vi "FinalizeScanSignals.vi"(8 "error in (no error)":errorcluster, 9 "Parameters":T1={"number of planes"=4, "z step"=1.9999999999999998e-05, "pixel dwell time"=1.0000000000000001e-11, "z frequency"=10.0, "number of pixels"=100, "smooth points"=10, "smooth line"=10, "Sine\nSawtooth"=FALSE, "PointSorting"=0, "Sort Points"=FALSE, "X-pixels"=256.0, "Y-lines"=256.0, "pixelstoµm"=256.0, "zoom"=1.0, "Time offset"=1.0000000000000001e-11} {"zoom" min=0.5 step=0.1; "Y-lines" min=1 step=1; "X-pixels" min=1 step=1; "PointSorting" items=["No Difference", "Every Second Point", "Down / Up"]; "smooth line" min=1; "smooth points" min=1; "number of pixels" min=1; "z frequency" format="%_4g"; "number of planes" min=1}, 10 "DutyCluster":T2 {"Iteration" items=["first iteration", "second iteration"]}, 11 "x pixels, y pixels, z, time":dbl[][](array[numeric])) -> (0 "error out":errorcluster, 3 "x (pixels), y (pixels), z (um), time (s)":dbl[][](array[numeric]))   [LabVIEW 2010]
uses:
  TypeDefs/DutyCluster.ctl
  TypeDefs/ParameterCluster.ctl
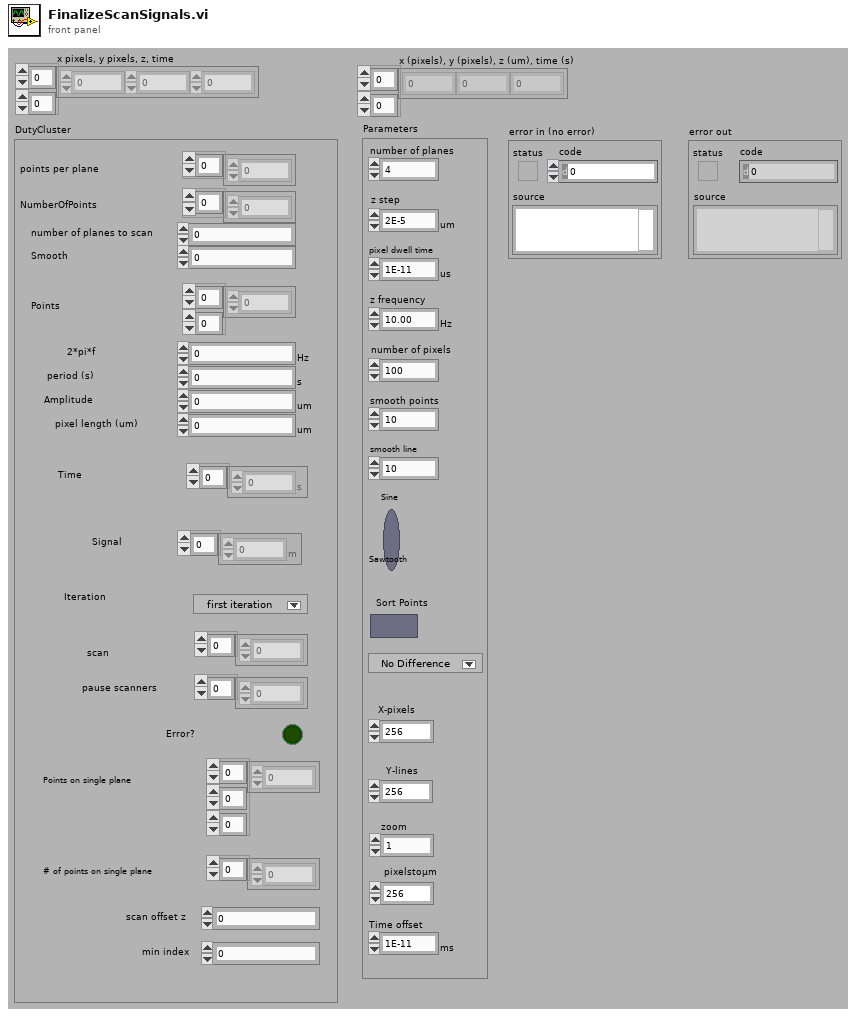
[diagram p1: front panel]
types:
  T1 = typedef "ParameterCluster.ctl" = cluster{"number of planes":i32, "z step":dbl[unit], "pixel dwell time":dbl[unit], "z frequency":dbl[unit], "number of pixels":i32, "smooth points":i32, "smooth line":i32, "Sine\nSawtooth":bool, "PointSorting":u16, "Sort Points":bool, "X-pixels":sgl, "Y-lines":sgl, "pixelstoµm":dbl, "zoom":dbl, "Time offset":dbl[unit]}
  T2 = typedef "DutyCluster.ctl" = cluster{"points per plane":i32[], "NumberOfPoints":i32[], "number of planes to scan":i32, "Smooth":i32, "Points":dbl[][], "2*pi*f":dbl[unit], "period (s)":dbl[unit], "Amplitude":dbl[unit], "pixel length (um)":dbl[unit], "Time":dbl[unit][], "Signal":dbl[unit][], "Iteration":u16, "scan":i32[], "pause scanners":i32[], "Error?":bool, "Points on single plane":dbl[][][], "# of points on single plane":i32[], "scan offset z":i32, "min index":i32}
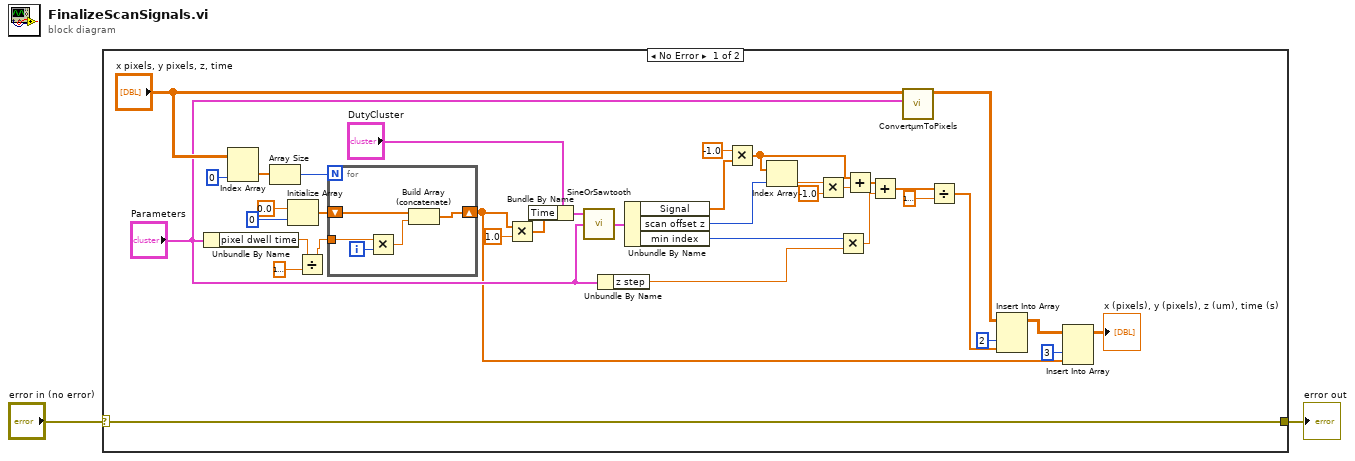
[diagram p0: block diagram]
diagram:
  n1 = case shown="No Error" "error in (no error)" {
    selector: "error in (no error)" -> [w10 w45]
    tunnel: [w10 w45] -> w1
    frame No Error {
      n2 = Unbundle By Name("Parameters") -> ("pixel dwell time"=w8:dbl[unit])
      n3 = Index Array(array="x pixels, y pixels, z, time", index (col)=0 ("disabled index (col)")) -> (element=w38:dbl[])  [unwired: 1 in]
      n4 = Array Size(array=w38) -> (size(s)=w34:i32)
      n5 = Initialize Array(0.0 ("element"), 0 ("dimension size")) -> (w35:dbl[])
      n6 = Divide(x=w8, y=dbl[unit] 1e-06) -> (x/y=w7:dbl)
      n7 = for {
        N: w34 -> [_]
        shift-right: [w40] -> w6
        shift-left: w35 -> [w41]
        tunnel: w7 -> [w43]
        i -> [w44]
        n8 = Multiply(x=w43, y=w44) -> (x*y=w42:dbl)
        n9 = Build Array (concatenate)(w41, w42) -> (w40:dbl[])
      }
      n10 = Multiply(x=w6, y=dbl[unit] 1.0) -> (x*y=w5:dbl[unit][])
      n11 = Bundle By Name(cluster="DutyCluster", "Time"=w5) -> (w32:T2)
      n12 = call "SineOrSawtooth.vi"("Parameters"="Parameters", "DutyCluster"=w32) -> ("DutyCluster"=w3:T2)  [unwired: 2 in, 1 out]
      n13 = Unbundle By Name("Parameters") -> ("z step"=w19:dbl[unit])
      n14 = Unbundle By Name(w3) -> ("Signal"=w20:dbl[unit][], "scan offset z"=w21:i32, "min index"=w18:i32)
      n15 = Multiply(x=-1.0 ("y"), y=w20) -> (x*y=w24:dbl[unit][])
      n16 = Index Array(array=w24, index=w21) -> (element=w28:dbl[unit])
      n17 = Multiply(x=w28, y=-1.0) -> (x*y=w26:dbl[unit])
      n18 = Multiply(x=w18, y=w19) -> (x*y=w23:dbl[unit])
      n19 = Add(x=w24, y=w26) -> (x+y=w22:dbl[unit][])
      n20 = Add(x=w22, y=w23) -> (x+y=w16:dbl[unit][])
      n21 = call "ConvertµmToPixels.vi"("Parameters"="Parameters", "Point coordinates (um)"="x pixels, y pixels, z, time") -> ("Point coordinates (pixels)"=w12:dbl[][])  [unwired: 8 in, 1 out]
      n22 = Divide(x=w16, y=dbl[unit] 1e-06) -> (x/y=w15:dbl[])
      n23 = Insert Into Array(array=w12, index (col)=2 ("disabled index (col)"), new element=w15) -> (w31:dbl[][])  [unwired: 1 in]
      n24 = Insert Into Array(array=w31, index (col)=3 ("disabled index (col)"), new element=w6) -> (→"x (pixels), y (pixels), z (um), time (s)":dbl[][])  [unwired: 1 in]
    }
    frame Error {
    }
  }
  "error out" <- w1
